vi "GetNodeMenuOptions.vi"(0 "reference in":refnum<class "DQMHModuleNode.lvclass">, 1 "MousePos":T1 {"y" format="%.2f"; "x" format="%.2f"}, 5 "error in (no error)":errorcluster) -> (14 "reference out":refnum<class "DQMHModuleNode.lvclass">, 15 "MenuOptions":string[](array[string]), 19 "error out":errorcluster)   [LabVIEW 2014, in "DQMHModuleNode.lvclass"]
doc: "Gets the menu option"
uses:
  <resource>/Framework/Providers/Open_GDS/UML/DQMHModuleNode_class/DQMHModuleNode.lvclass
  <resource>/Framework/Providers/Open_GDS/UML/General/Point/Point Point2D.ctl
  <resource>/Framework/Providers/Open_GDS/UML/RectangularNode_class/RectangularNode.lvclass
  <resource>/Framework/Providers/Open_GDS/UML/MultiLineString_class/MultiLineString.lvclass
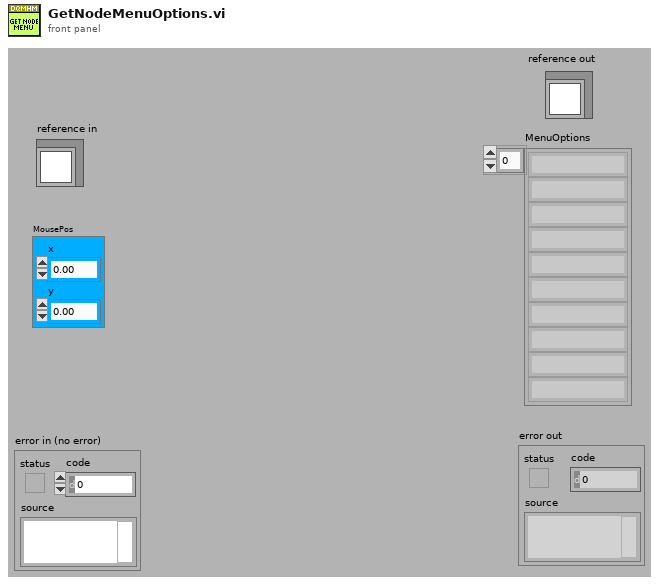
[diagram p1: front panel]
types:
  T1 = typedef "Point Point2D.ctl" = cluster{"x":dbl, "y":dbl}
  T2 = typedef "DQMHModuleNode.lvclass/ObjectAttributes.ctl" = cluster{"midHeight":dbl, "botHeight":dbl, "Name":refnum<class "MultiLineString.lvclass">, "Description":refnum<class "MultiLineString.lvclass">, "InternalData":refnum<class "MultiLineString.lvclass">, "Events":refnum<class "MultiLineString.lvclass">, "DEFAULT_COMPARTMENT_HEIGHT":i32, "DEFAULT_WIDTH":i32, "DEFAULT_HEIGHT":i32, "showEvents":bool, "showInternalData":bool, "ClassPath":path, "Template":string, "Icon":u8[][]}
  T3 = typedef "RectangularNode.lvclass/ObjectAttributes.ctl" = cluster{"bounds":T4}
  T4 = typedef "Rectangle Rectangle2D.ctl" = cluster{"x":dbl, "y":dbl, "width":dbl, "height":dbl}
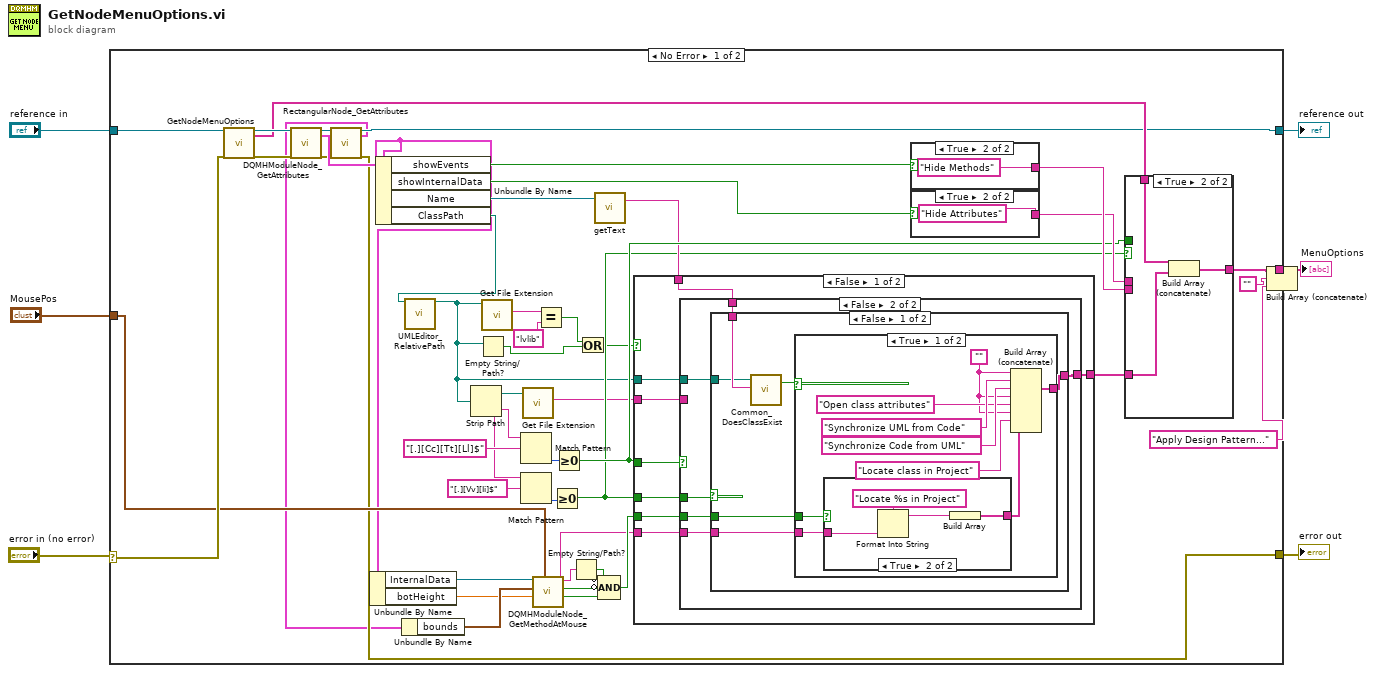
[diagram p0: block diagram]
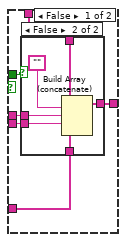
[diagram p2: hidden frame]
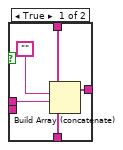
[diagram p3: hidden frame]
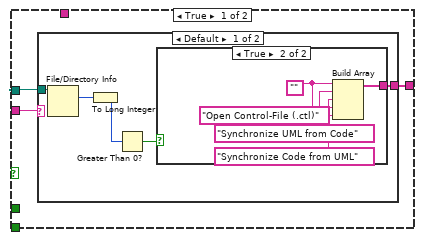
[diagram p4: hidden frame]
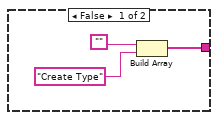
[diagram p5: hidden frame]
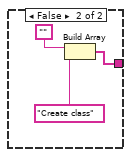
[diagram p8: hidden frame]
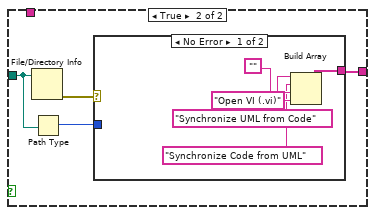
[diagram p9: hidden frame]
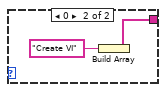
[diagram p11: hidden frame]
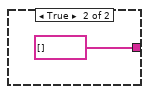
[diagram p12: hidden frame]
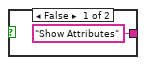
[diagram p13: hidden frame]
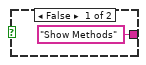
[diagram p14: hidden frame]
diagram:
  n1 = case shown="No Error" "error in (no error)" {
    selector: "error in (no error)" -> [w27 w144]
    tunnel: "reference in" -> [w28 w145]
    tunnel: [w9 w144] -> w5
    tunnel: [w8 w145] -> w4
    tunnel: [w15 _] -> w2
    tunnel: "MousePos" -> [w24 _]
    frame No Error {
      n2 = call-parent "GetNodeMenuOptions.vi"("reference"=w28, "error in (no error)"=w27) -> ("reference out"=w30:refnum<class "DQMHModuleNode.lvclass">, "MenuOptions"=w29:string[], "error out"=w26:errorcluster)  [unwired: 15 in]
      n3 = call <resource>:"DQMHModuleNode_GetAttributes.vi"("reference in"=w30, "error in (no error)"=w26) -> ("reference out"=w11:refnum<class "DQMHModuleNode.lvclass">, "Data"=w12:T2, "error out"=w10:errorcluster)  [unwired: 1 in, 14 out]
      n4 = call <resource>:"RectangularNode_GetAttributes.vi"("reference in"=w11, "error in (no error)"=w10) -> ("reference out"=w8:refnum<class "DQMHModuleNode.lvclass">, "Data"=w7:T3, "error out"=w9:errorcluster)  [unwired: 14 in, 1 out]
      n5 = Unbundle By Name(w12) -> ("InternalData"=w25:refnum<class "MultiLineString.lvclass">, "botHeight"=w22:dbl)
      n6 = Unbundle By Name(w12) -> ("showEvents"=w53:bool, "showInternalData"=w52:bool, "Name"=w45:refnum<class "MultiLineString.lvclass">, "ClassPath"=w43:path)
      n7 = Unbundle By Name(w7) -> ("bounds"=w23:T4)
      n8 = call <resource>:"UMLEditor_RelativePath.vi"("Path In"=w43) -> ("ConvertToAbsolutePath(If possible)"=w38:path)  [unwired: 1 in, 17 out]
      n9 = Strip Path(path=w38) -> (stripped path=w32:path, name=w42:string)
      n10 = Empty String/Path?(string/path=w38) -> (empty?=w34:bool)
      n11 = call <vilib>:"Get File Extension.vi"("file"=w38) -> ("lowercase file extension"=w37:string)  [unwired: 1 in, 9 out]
      n12 = Match Pattern(string=w42, regular expression="[.][Cc][Tt][Ll]$") -> (offset past match=w47:i32)  [unwired: 4 out]
      n13 = Match Pattern(string=w42, regular expression="[.][Vv][Ii]$") -> (offset past match=w40:i32)  [unwired: 4 out]
      n14 = call <vilib>:"Get File Extension.vi"("file"=w32) -> ("lowercase file extension"=w31:string)  [unwired: 1 in, 9 out]
      n15 = call <resource>:"DQMHModuleNode_GetMethodAtMouse.vi"("MousePos"=w24, "botHeight"=w22, "bounds"=w23, "reference in"=w25) -> ("MethodSelected"=w20:bool, "NoMmethodsExists"=w21:bool, "MEthodName"=w17:string)  [unwired: 2 in, 1 out]
      n16 = Equal?(x=w37, y="lvlib") -> (x = y?=w33:bool)
      n17 = Greater Or Equal To 0?(x=w40) -> (x >= 0?=w39:bool)
      n18 = Greater Or Equal To 0?(x=w47) -> (x >= 0?=w46:bool)
      n19 = Empty String/Path?(string/path=w17) -> (empty?=w19:bool)
      n20 = Or(x=w33, y=w34) -> (x .or. y?=w35:bool)
      n21 = call-dynamic "getText.vi"("reference"=w45) -> ("text"=w44:string)  [unwired: 16 in, 2 out]
      n22 = Compound Arithmetic op=AND(invert w19, invert w21, w20) -> (w18:bool)
      n23 = case shown="False" w35 {
        tunnel: [w81 string[] []] -> w51
        tunnel: w46 -> [w80 _]
        tunnel: w38 -> [w79 _]
        tunnel: w44 -> [w78 _]
        tunnel: w39 -> [w77 _]
        tunnel: w31 -> [w76 _]
        tunnel: w18 -> [w75 _]
        tunnel: w17 -> [w74 _]
        frame False {
          n24 = case shown="False" w80 {
            tunnel: [w84 w103] -> w81
            tunnel: w79 -> [w83 w101]
            tunnel: w78 -> [_ w102]
            tunnel: w77 -> [_ w100]
            tunnel: w76 -> [w82 _]
            tunnel: w75 -> [_ w99]
            tunnel: w74 -> [_ w98]
            frame True {
              n25 = case shown="Default" w82 {
                tunnel: [w89 _] -> w84
                tunnel: w83 -> [w87 _]
                frame Default {
                  n26 = File/Directory Info(path=w87) -> (size=w85:i64)  [unwired: 1 in, 6 out]
                  n27 = To Long Integer(number=w85) -> (32bit integer=w88:i32)
                  n28 = Greater Than 0?(x=w88) -> (x > 0?=w86:bool)
                  n29 = case shown="True" w86 {
                    tunnel: [w91 w97] -> w89
                    frame False {
                      n30 = Build Array("", "Create Type" ("element")) -> (w91:string[])
                    }
                    frame True {
                      w94 = ""
                      n31 = Build Array(w94, "Synchronize UML from Code" ("element"), "Synchronize Code from UML" ("element"), w94, "Open Control-File (.ctl)" ("element")) -> (w97:string[])
                    }
                  }
                }
                frame "lvclass" {
                }
              }
            }
            frame False {
              n32 = case shown="False" w100 {
                tunnel: [w109 w129] -> w103
                tunnel: w102 -> [w108 _]
                tunnel: w101 -> [w106 w127]
                tunnel: w99 -> [w105 _]
                tunnel: w98 -> [w104 _]
                frame False {
                  n33 = call <resource>:"Common_DoesClassExist.vi"("ClassPath"=w106, "ClassName"=w108) -> ("ClassExists"=w107:bool)  [unwired: 17 out]
                  n34 = case shown="True" w107 {
                    tunnel: [w118 w125] -> w109
                    tunnel: w105 -> [w112 _]
                    tunnel: w104 -> [w111 _]
                    frame True {
                      w114 = ""
                      n35 = case shown="True" w112 {
                        tunnel: w111 -> [_ w122]
                        tunnel: [_ w119] -> w110
                        frame False {
                        }
                        frame True {
                          n36 = Format Into String(format string="Locate %s in Project" ("element"), w122) -> (resulting string=w120:string)  [unwired: 2 in, 1 out]
                          n37 = Build Array(w120) -> (w119:string[])
                        }
                      }
                      n38 = Build Array (concatenate)(w114, "Synchronize UML from Code" ("element"), "Synchronize Code from UML" ("element"), w114, "Open class attributes" ("element"), w114, "Locate class in Project" ("element"), w110) -> (w118:string[])
                    }
                    frame False {
                      n39 = Build Array("", "Create class" ("element")) -> (w125:string[])
                    }
                  }
                }
                frame True {
                  n40 = File/Directory Info(path=w127) -> (error out=w128:errorcluster)  [unwired: 1 in, 6 out]
                  n41 = Path Type(1:w127) -> (0:w126:i16)
                  n42 = case shown="No Error" w128 {
                    tunnel: [w134 w136] -> w129
                    tunnel: w126 -> [_ w135]
                    frame No Error {
                      n43 = Build Array("Synchronize UML from Code" ("element"), "Synchronize Code from UML" ("element"), "", "Open VI (.vi)" ("element")) -> (w134:string[])
                    }
                    frame Error {
                      n44 = case shown="Default" w135 {
                        tunnel: [_ w138] -> w136
                        frame Default {
                        }
                        frame 0 {
                          n45 = Build Array("Create VI" ("element")) -> (w138:string[])
                        }
                      }
                    }
                  }
                }
              }
            }
          }
        }
        frame True {
        }
      }
      n46 = case shown="True" w53 {
        tunnel: ["Show Methods" "Hide Methods"] -> w50
        frame False {
        }
        frame True {
        }
      }
      n47 = case shown="True" w52 {
        tunnel: ["Show Attributes" "Hide Attributes"] -> w49
        frame False {
        }
        frame True {
        }
      }
      n48 = case shown="True" w39 {
        tunnel: [w59 w73] -> w16
        tunnel: w51 -> [w58 w72]
        tunnel: w50 -> [w57 _]
        tunnel: w49 -> [w56 _]
        tunnel: w46 -> [w55 _]
        tunnel: w29 -> [w54 w71]
        frame False {
          n49 = case shown="False" w55 {
            tunnel: [w64 w70] -> w59
            tunnel: w58 -> [w61 w68]
            tunnel: w57 -> [_ w67]
            tunnel: w56 -> [w62 w66]
            tunnel: w54 -> [w60 w65]
            frame True {
              n50 = Build Array (concatenate)(w60, "", w62, w61) -> (w64:string[])
            }
            frame False {
              n51 = Build Array (concatenate)(w65, "", w66, w67, w68) -> (w70:string[])
            }
          }
        }
        frame True {
          n52 = Build Array (concatenate)(w71, w72) -> (w73:string[])
        }
      }
      n53 = Build Array (concatenate)(w16, "", "Apply Design Pattern..." ("element")) -> (w15:string[])
    }
    frame Error {
    }
  }
  "reference out" <- w4
  "error out" <- w5
  "MenuOptions" <- w2
